vi "SwerveShortestTurnAlg.vi"(7 "Z":dbl, 8 "SwerveMotorsFlipped?":bool, 9 "SwerveSpeed":dbl, 10 "AngleSetpoint":dbl, 11 "AngleEncoder":dbl) -> (2 "FlipSwerveMotors":bool, 3 "PIDInput":dbl)   [LabVIEW 2019]
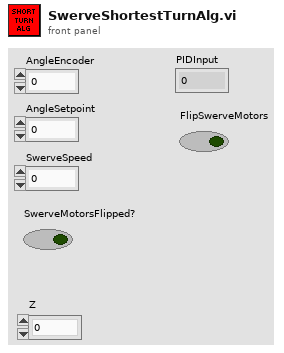
[diagram p1: front panel]
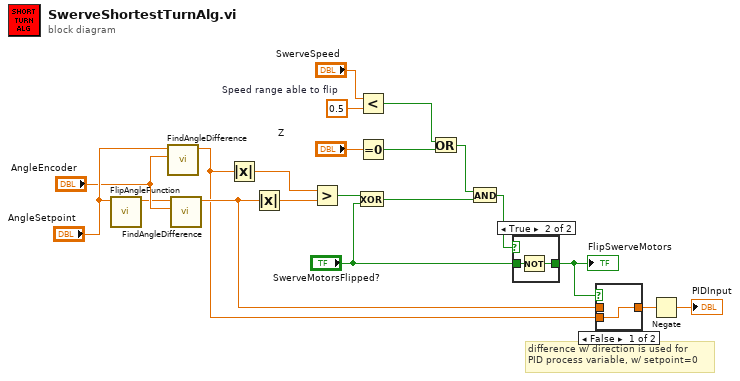
[diagram p0: block diagram]
diagram:
  w12 = 0.5  # Speed range able to flip
  # "difference w/ direction is used for\nPID process variable, w/ setpoint=0"
  n1 = call "FlipAngleFunction.vi"("AngleInput"="AngleSetpoint") -> ("AngleFlipped"=w14:dbl)  [unwired: 10 in]
  n2 = call "FindAngleDifference.vi"("AngleEncoder"="AngleEncoder", "AngleSetpoint"="AngleSetpoint") -> ("Distance/DirectionOfTurn"=w13:dbl)  [unwired: 9 in]
  n3 = call "FindAngleDifference.vi"("AngleEncoder"="AngleEncoder", "AngleSetpoint"=w14) -> ("Distance/DirectionOfTurn"=w15:dbl)  [unwired: 9 in]
  n4 = Absolute Value(x=w13) -> (abs(x)=w8:dbl)
  n5 = Absolute Value(x=w15) -> (abs(x)=w7:dbl)
  n6 = Greater?(x=w8, y=w7) -> (0:w10:bool)
  n7 = Exclusive Or(1:"SwerveMotorsFlipped?", 2:w10) -> (0:w6:bool)
  n8 = Less?(x="SwerveSpeed", y=w12) -> (x < y?=w2:bool)
  n9 = Equal To 0?(x="Z") -> (x = 0?=w1:bool)
  n10 = Or(x=w2, y=w1) -> (x .or. y?=w5:bool)
  n11 = And(x=w5, y=w6) -> (x .and. y?=w3:bool)
  n12 = case shown="True" w3 {
    tunnel: "SwerveMotorsFlipped?" -> [w21 w23]
    tunnel: [w21 w22] -> w17
    frame False {
    }
    frame True {
      n13 = Not(x=w23) -> (.not. x?=w22:bool)
    }
  }
  "FlipSwerveMotors" <- w17
  n14 = case shown="False" w17 {
    tunnel: w13 -> [w24 _]
    tunnel: w15 -> [_ w25]
    tunnel: [w24 w25] -> w16
    frame False {
    }
    frame True {
    }
  }
  n15 = Negate(x=w16) -> (-x=→"PIDInput":dbl)
